vi "Check Errors.vi"(8 "error in (no error)":errorcluster, 11 "Session in":refnum<class "Session.lvclass">) -> (0 "error out":errorcluster, 3 "Session out":refnum<class "Session.lvclass">)   [LabVIEW 2020, in "CTI.lvlib" / "Session.lvclass"]
doc: "Queries the device for any errors that have been queued by the firmware. If the device supports queuing multiple errors and several have been generated, they will all be reported in a single error value."
uses:
  Session.lvclass
  DeviceComms/DeviceComms.lvclass
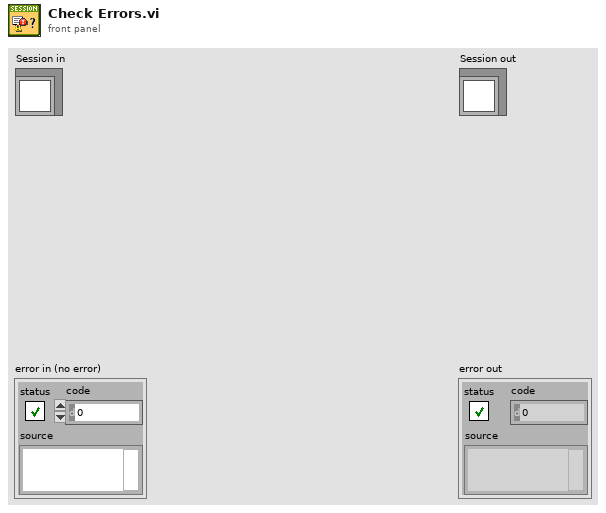
[diagram p1: front panel]
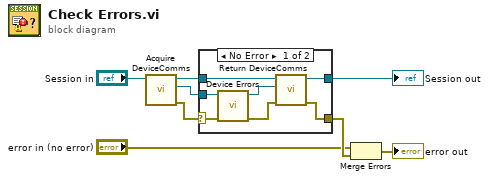
[diagram p0: block diagram]
diagram:
  n1 = call "Acquire DeviceComms.vi"("Session in"="Session in") -> ("error out"=w6:errorcluster, "DeviceComms"=w7:refnum<class "DeviceComms.lvclass">, "Session out"=w5:refnum<class "Session.lvclass">)  [unwired: 8 in]
  n2 = case shown="No Error" w6 {
    selector: w6 -> [w14 w17]
    tunnel: w7 -> [w15 _]
    tunnel: w5 -> [w13 w16]
    tunnel: [w10 w16] -> w4
    tunnel: [w9 w17] -> w3
    frame No Error {
      n3 = call-dynamic "Device Errors.vi"("error in (no error)"=w14, "DeviceComms in"=w15) -> ("error out"=w11:errorcluster, "DeviceComms out"=w12:refnum<class "DeviceComms.lvclass">)  [unwired: 8 in]
      n4 = call "Return DeviceComms.vi"("error in (no error)"=w11, "DeviceComms"=w12, "Session in"=w13) -> ("error out"=w9:errorcluster, "Session out"=w10:refnum<class "Session.lvclass">)  [unwired: 7 in]
    }
    frame Error {
    }
  }
  "Session out" <- w4
  n5 = Merge Errors("error in (no error)", w3) -> (→"error out":errorcluster)
